vi "Export Image.vi"(7 "Temporary Image Directory":path, 8 "Error in":errorcluster caption="Error in (no error)", 10 "Image Data":T1, 11 "Name":string) -> (0 "Error out":errorcluster, 3 "Image Path":path)   [LabVIEW 2023, in "VIDoc Printer.lvlib" / "VIDoc Printer.lvclass"]
doc: "Exports Image Data as a png file stored in the Temporary Image Directory"
uses:
  VIDoc Printer.lvclass
  <vilib>/picture/picture.llb/imagedata.ctl
  <vilib>/Utility/error.llb/DialogType.ctl
  VIDoc Printer.lvclass/VIDoc Printer.ctl
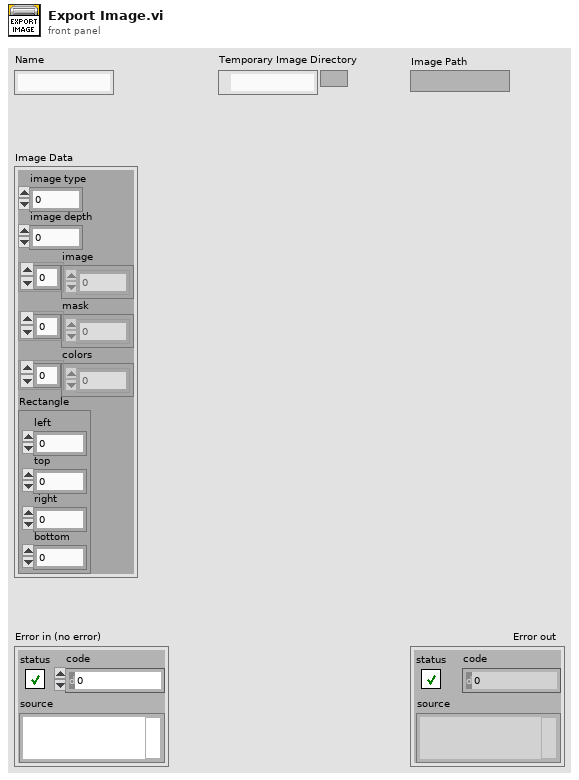
[diagram p1: front panel]
types:
  T1 = typedef "imagedata.ctl" = cluster{"image type":i32, "image depth":i32, "image":u8[], "mask":u8[], "colors":u32[], "Rectangle":cluster{"left":i16, "top":i16, "right":i16, "bottom":i16}}
  T2 = typedef "DialogType.ctl" = u16
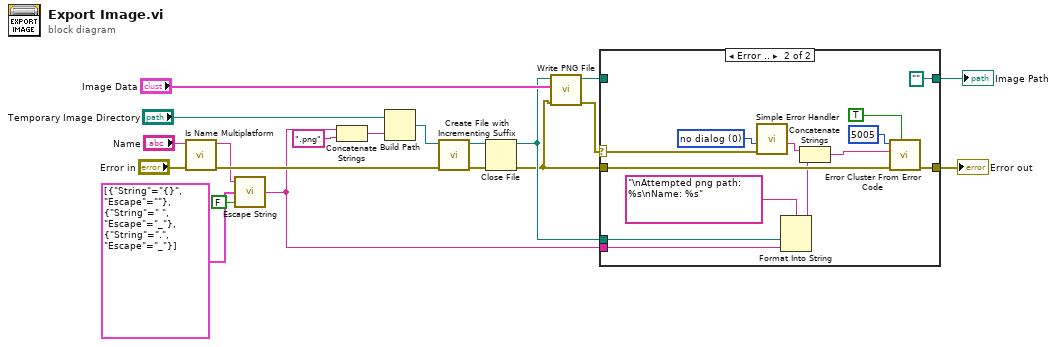
[diagram p0: block diagram]
diagram:
  n1 = call <vilib>:"Is Name Multiplatform.vi"("error in (no error)"="Error in", "filename"="Name") -> ("error out"=w10:errorcluster, "suggested filename"=w3:string)  [unwired: 5 in, 3 out]
  n2 = call <vilib>:"Escape String.vi"("Remove Escapes? (False)"=FALSE, "Escapes"=cluster{"String":string, "Escape":string}[] [{"String"="{}", "Escape"=""}, {"String"=" ", "Escape"="_"}, {"String"=".", "Escape"="_"}], "String in"=w3) -> ("String out"=w2:string)
  n3 = Concatenate Strings(w2, ".png" ("string")) -> (w14:string)
  n4 = Build Path(base path="Temporary Image Directory", name or relative path=w14) -> (appended path=w9:path)
  n5 = call <vilib>:"Create File with Incrementing Suffix.vi"("error in (no error)"=w10, "file path"=w9) -> ("error out"=w8:errorcluster, "refnum out"=w7:refnum<file>)  [unwired: 7 in, 1 out]
  n6 = Close File(refnum=w7, error in=w8) -> (path=w6:path, error out=w5:errorcluster)
  n7 = call <vilib>:"Write PNG File.vi"("error in (no error)"=w5, "image data"="Image Data", "path to PNG file"=w6) -> ("error out"=w18:errorcluster, "path"=w11:path)  [unwired: 7 in]
  n8 = case shown="Error .." w18 {
    selector: w18 -> [_ w32]
    tunnel: [w22 w29] -> w17
    tunnel: w5 -> [w22 w28]
    tunnel: w6 -> [_ w26]
    tunnel: w2 -> [_ w25]
    tunnel: [w21 path ""] -> w12
    tunnel: w11 -> [w21 _]
    frame No Error {
    }
    frame Error {
      w33 = T2 0 items=["no dialog", "OK message", "continue or stop message", "OK message + warnings", "continue/stop + warnings"] ("type of dialog (OK msg:1)")
      n9 = call <vilib>:"Simple Error Handler.vi"("type of dialog (OK msg:1)"=w33, "error in (no error)"=w32) -> ("source out"=w31:string)  [unwired: 3 in, 4 out]
      n10 = Format Into String(format string="\nAttempted png path: %s\nName: %s", w26, w25) -> (resulting string=w24:string)  [unwired: 2 in, 1 out]
      n11 = Concatenate Strings(w31, w24) -> (w30:string)
      n12 = call <vilib>:"Error Cluster From Error Code.vi"("show call chain? (False)"=TRUE, "error in (no error)"=w28, "error message (\"\")"=w30, "error code (0)"=5005) -> ("error out"=w29:errorcluster)  [unwired: 5 in]
    }
  }
  "Error out" <- w17
  "Image Path" <- w12
